vi "Batch Distillation.vi"() -> ()   [LabVIEW 2017]
uses:
  Reflux BatchD.vi
  Halt BatchD.vi
panel:
  out "Reboiler Temperature":dbl format="%#_3g"
  in  "Reflux Ratio":dbl
  in  "Reflux Control":bool
  in  "Main Power Switch":bool
  in  "Reboiler Power Switch":bool
  in  "stop":bool
  out "Data Point Count":i32
  in  "Specify Time between Data Points (sec)":dbl=1.0
  in  "Cancel Data Collection":bool
  in  "Specify number of data points":i16=1
  in  "Enable 4":bool
  out "Saving Data 4":bool
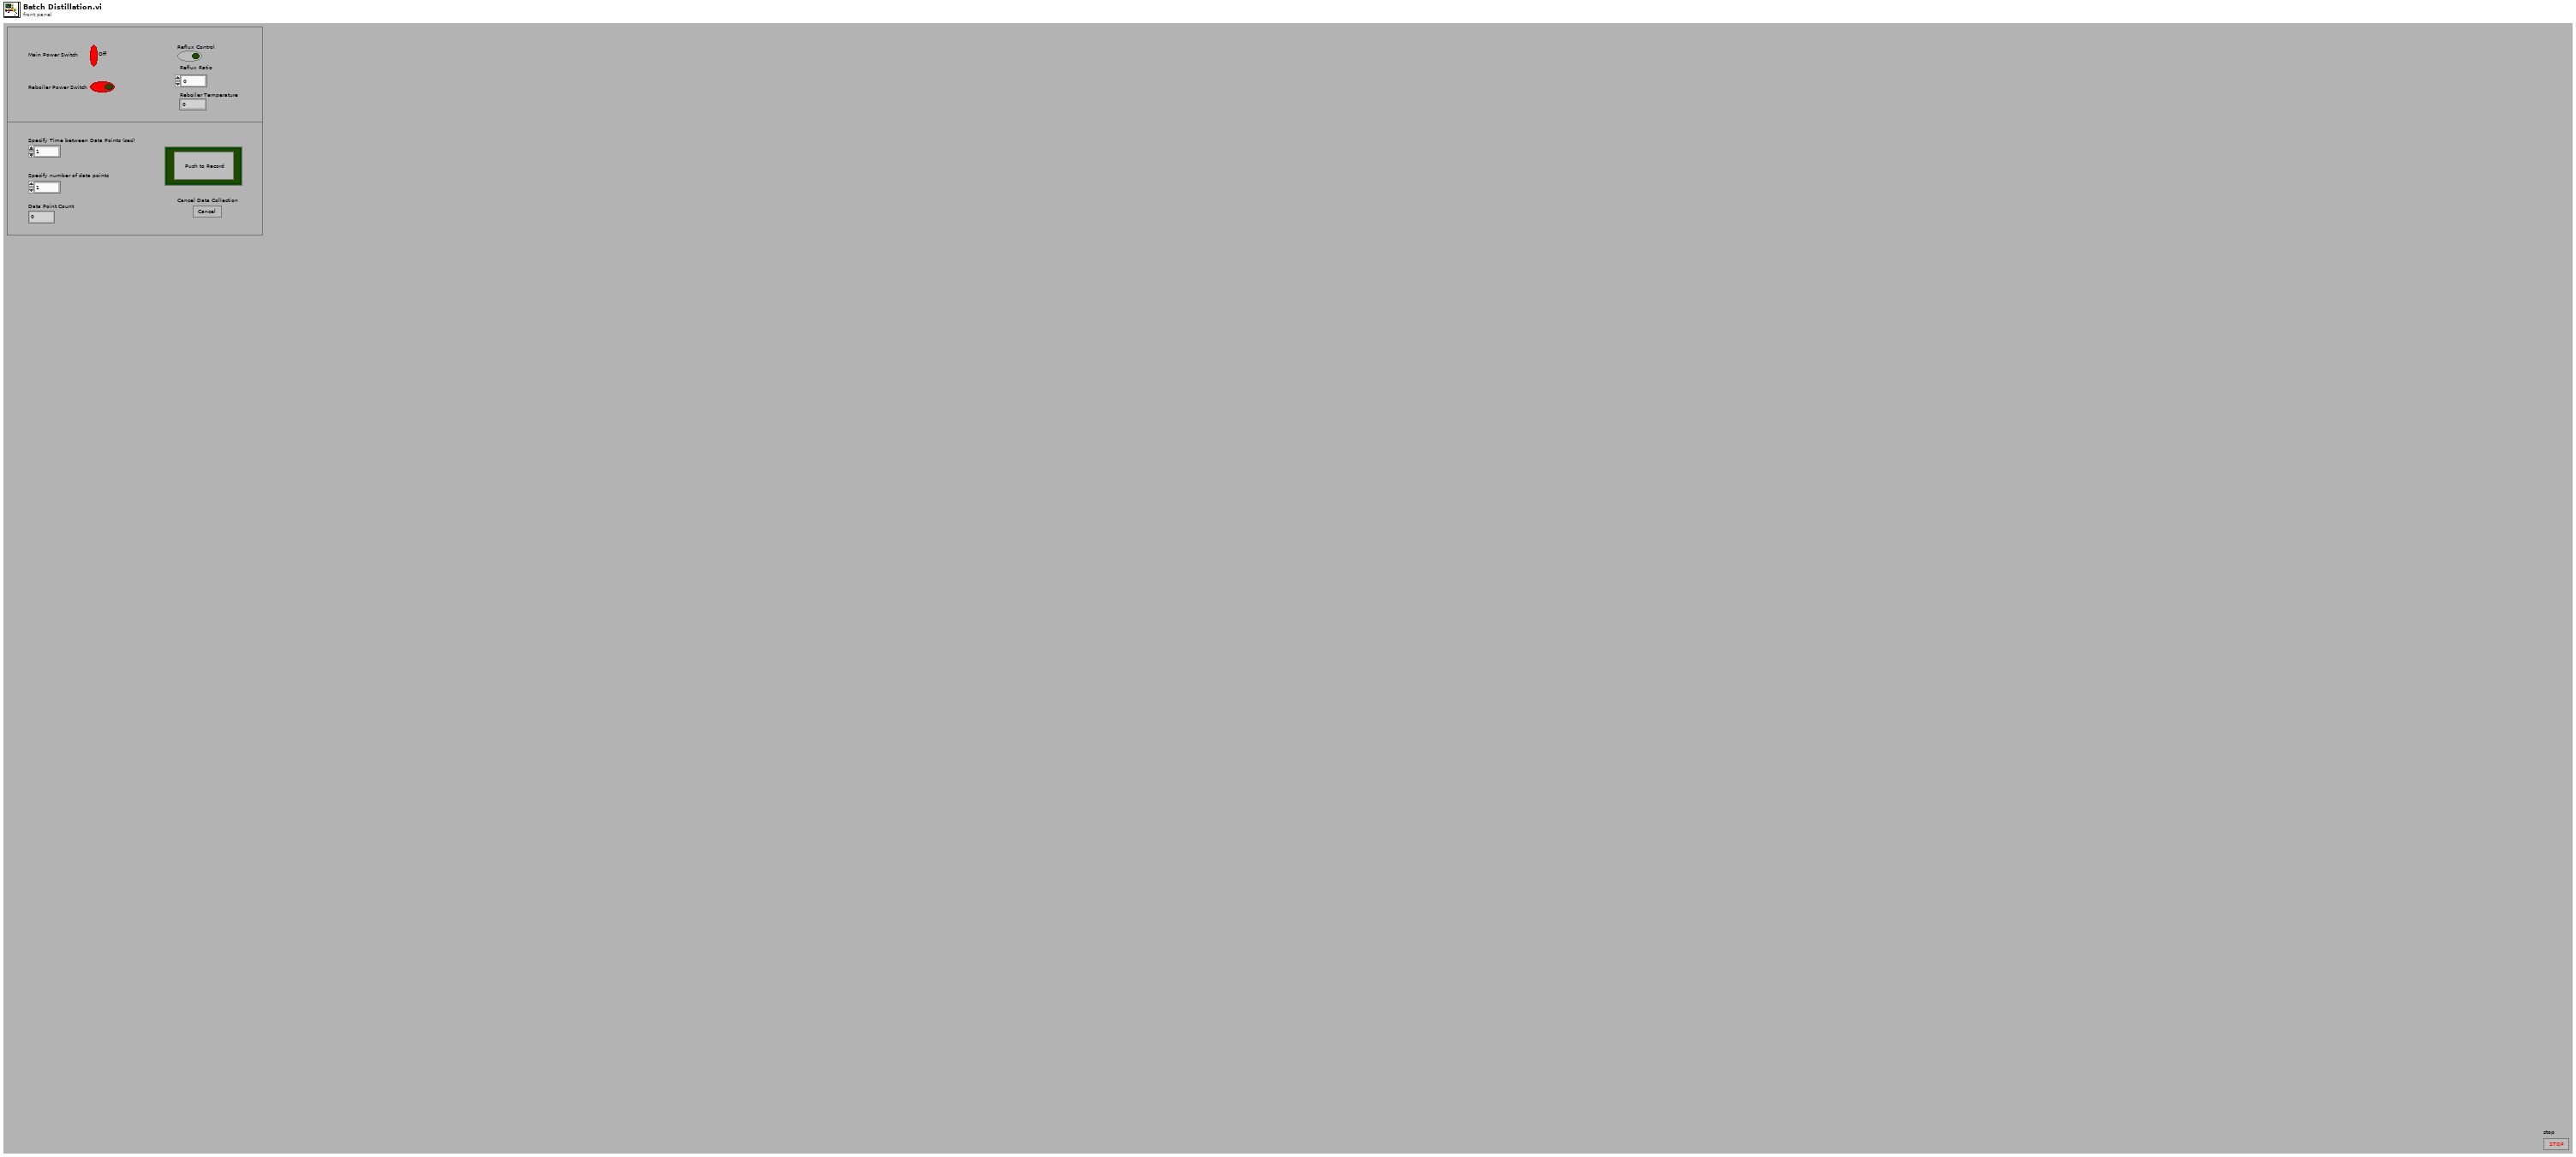
[diagram p1: front panel]
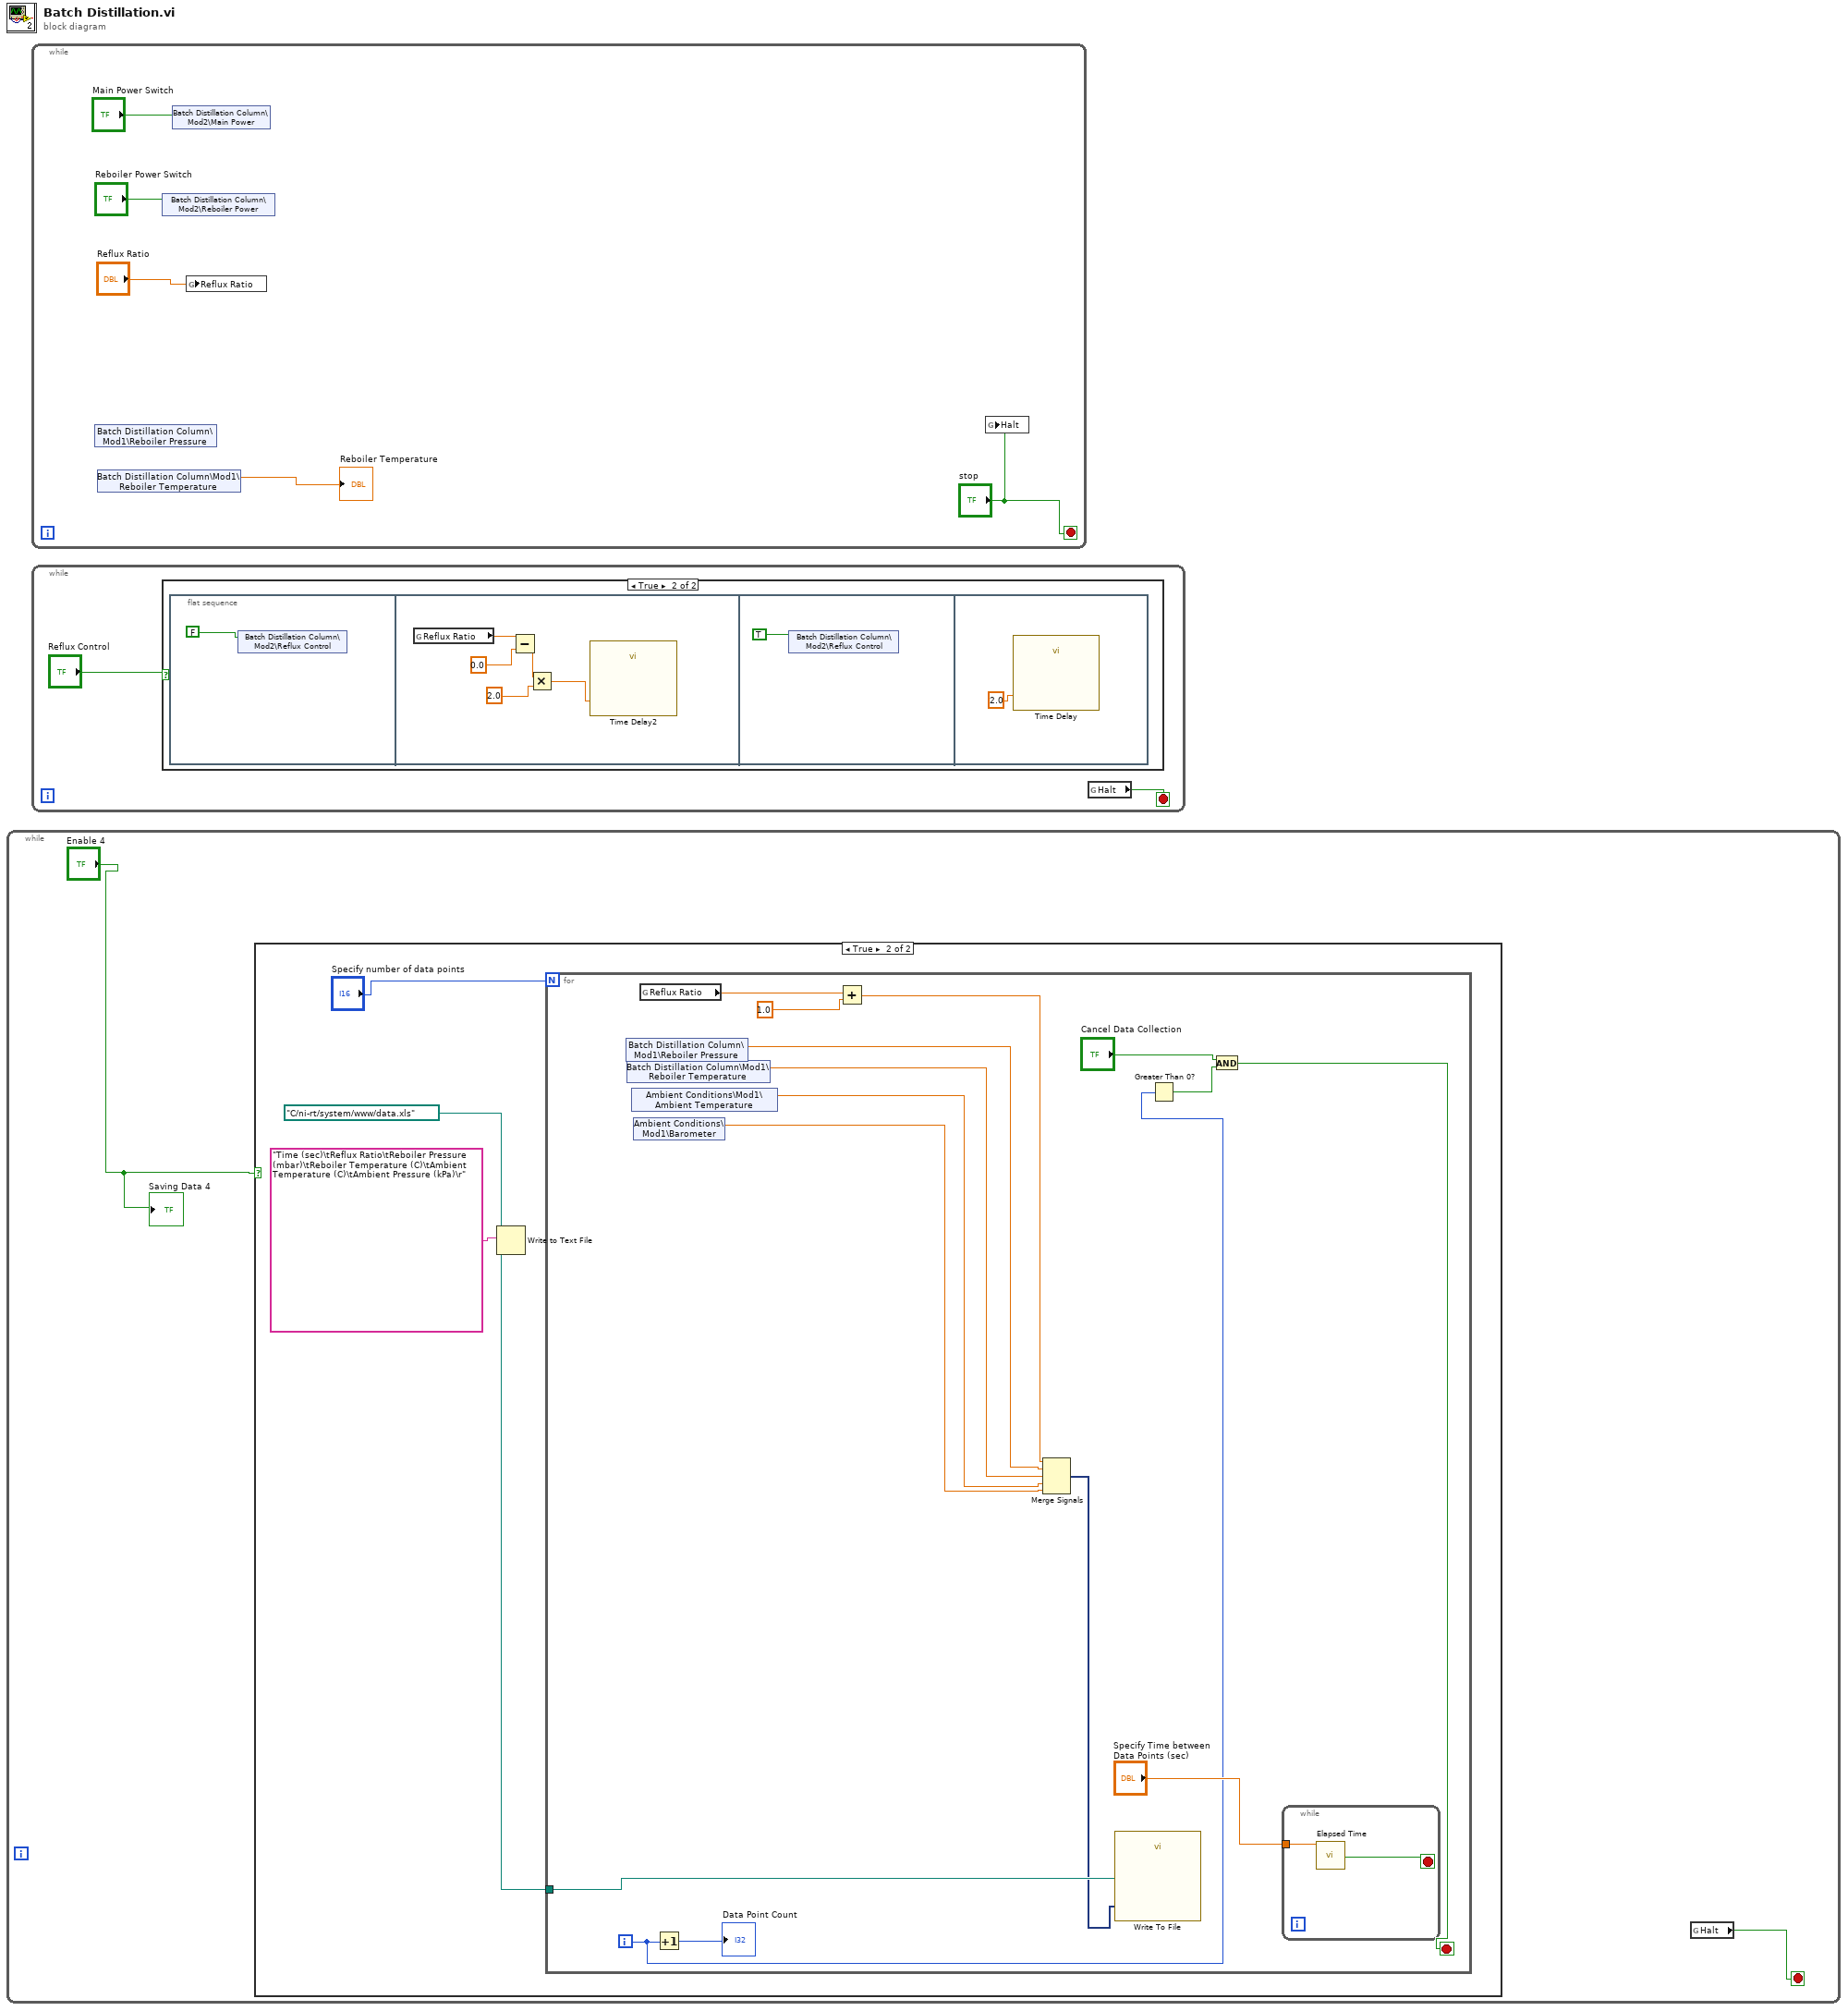
[diagram p0: block diagram]
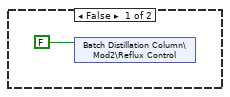
[diagram p2: hidden frame]
diagram:
  n1 = while {
    stop <- w1 stop-if-true
    n2 = case shown="True" "Enable 4" {
      frame False {
      }
      frame True {
        w4 = path "C:/ni-rt/system/www/data.xls" ("Filename")
        n3 = Write to Text File(file (use dialog)=w4, text="Time (sec)\tReflux Ratio\tReboiler Pressure (mbar)\tReboiler Temperature (C)\tAmbient Temperature (C)\tAmbient Pressure (kPa)\r") -> ()  [unwired: 2 in, 3 out]
        n4 = for {
          N: "Specify number of data points" -> [_]
          tunnel: w4 -> [w20]
          i -> [w16]
          stop <- w13 stop-if-true
          n5 = shared-variable "Batch Distillation Column\\Mod1\\Reboiler Pressure"() -> (w12:dbl)  [unwired: 1 in, 1 out]
          n6 = shared-variable "Batch Distillation Column\\Mod1\\Reboiler Temperature"() -> (w11:dbl)  [unwired: 1 in, 1 out]
          n7 = shared-variable "Ambient Conditions\\Mod1\\Ambient Temperature"() -> (w10:dbl)  [unwired: 1 in, 1 out]
          n8 = shared-variable "Ambient Conditions\\Mod1\\Barometer"() -> (w9:dbl)  [unwired: 1 in, 1 out]
          n9 = global read "Reflux BatchD.vi" "Reflux Ratio"() -> (w7:dbl)
          n10 = Increment(x=w16) -> (x+1=→"Data Point Count":i32)
          n11 = Add(x=w7, y=1.0) -> (x+y=w6:dbl)
          n12 = Merge Signals(w6, w12, w11, w10, w9) -> (w18:dynamicdata)
          n13 = call "Write To File"("Signals"=w18, "Filename"=w20) -> ()  [unwired: 15 in, 3 out]
          n14 = Greater Than 0?(x=w16) -> (x > 0?=w14:bool)
          n15 = And(x="Cancel Data Collection", y=w14) -> (x .and. y?=w13:bool)
          n16 = while {
            tunnel: "Specify Time between Data Points (sec)" -> [w21]
            stop <- w22 stop-if-true
            n17 = call "Elapsed Time"("Time Target (s)"=w21) -> ("Time has Elapsed"=w22:bool)  [unwired: 11 in, 7 out]
          }
        }
      }
    }
    n18 = global read "Halt BatchD.vi" "Halt"() -> (w1:bool)
    "Saving Data 4" <- "Enable 4"
  }
  n19 = while {
    stop <- "stop" stop-if-true
    n20 = shared-variable "Batch Distillation Column\\Mod1\\Reboiler Pressure"() -> ()  [unwired: 1 in, 2 out]
    n21 = shared-variable "Batch Distillation Column\\Mod1\\Reboiler Temperature"() -> (→"Reboiler Temperature":dbl)  [unwired: 1 in, 1 out]
    n22 = shared-variable "Batch Distillation Column\\Mod2\\Reboiler Power"("Reboiler Power Switch") -> ()  [unwired: 1 in, 1 out]
    n23 = shared-variable "Batch Distillation Column\\Mod2\\Main Power"("Main Power Switch") -> ()  [unwired: 1 in, 1 out]
    n24 = global write "Reflux BatchD.vi" "Reflux Ratio"("Reflux Ratio") -> ()
    n25 = global write "Halt BatchD.vi" "Halt"("stop") -> ()
  }
  n26 = while {
    stop <- w29 stop-if-true
    n27 = case shown="True" "Reflux Control" {
      frame False {
        n28 = shared-variable "Batch Distillation Column\\Mod2\\Reflux Control"(FALSE) -> ()  [unwired: 1 in, 1 out]
      }
      frame True {
        n29 = flat-sequence {
          frame #0 {
            n30 = shared-variable "Batch Distillation Column\\Mod2\\Reflux Control"(FALSE) -> ()  [unwired: 1 in, 1 out]
          }
          frame #1 {
            n31 = global read "Reflux BatchD.vi" "Reflux Ratio"() -> (w35:dbl)
            n32 = Subtract(x=w35, y=0.0) -> (x-y=w34:dbl)
            n33 = Multiply(x=w34, y=2.0) -> (x*y=w32:dbl)
            n34 = call "Time Delay2"("Delay Time (s)"=w32) -> ()  [unwired: 10 in, 1 out]
          }
          frame #2 {
            n35 = shared-variable "Batch Distillation Column\\Mod2\\Reflux Control"(TRUE) -> ()  [unwired: 1 in, 1 out]
          }
          frame #3 {
            n36 = call "Time Delay"("Delay Time (s)"=2.0) -> ()  [unwired: 10 in, 1 out]
          }
        }
      }
    }
    n37 = global read "Halt BatchD.vi" "Halt"() -> (w29:bool)
  }
